vi "Init Runtime.vi"(8 "error in (no error)":errorcluster, 10 "data allocations":T1, 11 "Numeric Limit Compare Config in":refnum<class "Numeric Limit Compare Config.lvclass">) -> (0 "error out":errorcluster, 2 "Skip":bool, 3 "Numeric Limit Compare Config out":refnum<class "Numeric Limit Compare Config.lvclass">)   [LabVIEW 2015, in "Numeric Limit Compare Config.lvclass"]
uses:
  Numeric Limit Compare Config.lvclass
  <vilib>/NI/Tag Bus Module Framework/channel/data tables.ctl
  <vilib>/NI/Tag Bus/dictionary/data dictionary.lvclass
  <vilib>/NI/Tag Bus/dictionary table pair.ctl
  <vilib>/NI/Tag Bus/table/data table.ctl
  Runtime/Numeric Limit Compare.lvclass
  Numeric Limit Compare Config.lvclass/Numeric Limit Compare Config.ctl
  <vilib>/NI/Tag Bus/tag/tag descriptor.lvclass/tag descriptor.ctl
  Runtime/Numeric Limit Compare.lvclass/Numeric Limit Compare.ctl
  Read Channel.vi
  Read Comparison Type.vi
  Read Upper Limit_Limit.vi
  Read Lower Limit.vi
  Read Negate Result.vi
  Read Result Channel.vi
  Runtime/Write Test Value Index.vi
  Runtime/Write Comparison Type.vi
  Runtime/Write Upper limit_limit.vi
  Runtime/Write Lower limit.vi
  Runtime/Write Negate Result.vi
  Runtime/Write Result Index.vi
  <vilib>/NI/Tag Bus/tag/read tag name.vi
  <vilib>/NI/Tag Bus/tag/read data type.vi
  <vilib>/NI/Tag Bus/dictionary/locate tag.vi
  <vilib>/NI/Tag Bus Module Framework/channel/TBM channel.lvclass
  <vilib>/NI/Tag Bus/table/data table.lvlib
  <vilib>/NI/Tag Bus/tag bus.lvlib
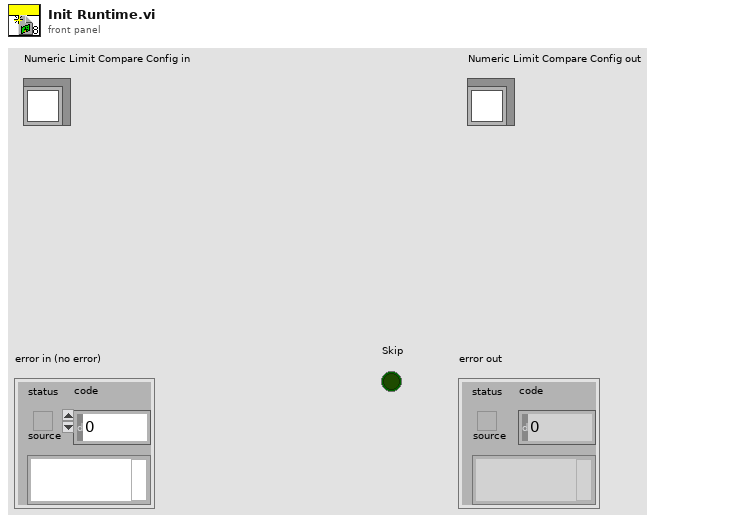
[diagram p1: front panel]
types:
  T1 = typedef "TBM channel.lvclass/data tables.ctl" = cluster{"input data":T2, "processing parameter":T2, "processing result":T2, "output data":T2}
  T2 = typedef "tag bus.lvlib/dictionary table pair.ctl" = cluster{"data dictionary":refnum<class "data dictionary.lvclass">, "data table":T3}
  T3 = typedef "tag bus.lvlib/data table.lvlib/data table.ctl" = cluster{"Double":dbl[], "Single":sgl[], "I64":i64[], "I32":i32[], "I16":i16[], "I8":i8[], "U64":u64[], "U32":u32[], "U16":u16[], "U8":u8[], "Boolean":bool[], "String":string[], "Array of Double":cluster{"DBL Array":dbl[]}[], "Array of Single":cluster{"SGL Array":sgl[]}[], "Array of I64":cluster{"I64 Array":i64[]}[], "Array of I32":cluster{"I32 Array":i32[]}[], "Array of I16":cluster{"I16 Array":i16[]}[], "Array of I8":cluster{"I8 Array":i8[]}[], "Array of U64":cluster{"U64 Array":u64[]}[], "Array of U32":cluster{"U32 Array":u32[]}[], "Array of U16":cluster{"U16 Array":u16[]}[], "Array of U8":cluster{"U8 Array":u8[]}[], "Array of Boolean":cluster{"Boolean Array":bool[]}[], "Array of String":cluster{"String Array":string[]}[]}
  T4 = typedef "Comparison Types.ctl" = enum16{"GELE (>=<=)", "GTLE(><=)", "GTLT(><)", "GELT(>=<)", "EQ(==)", "NE (!=)", "GT(>)", "LT(<)", "GE(>=)", "LE(<=)"}
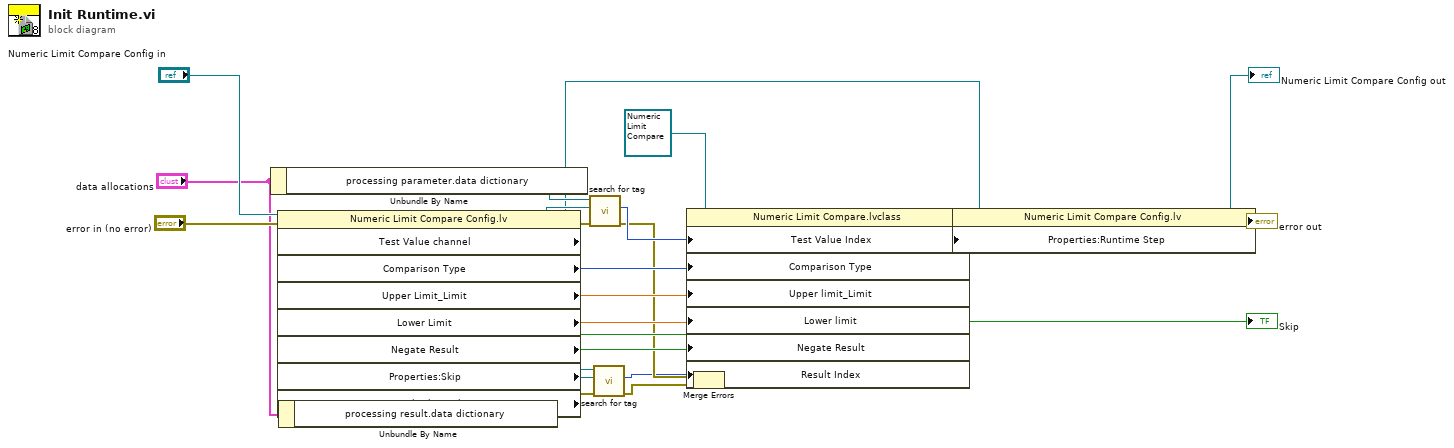
[diagram p0: block diagram]
diagram:
  n1 = Unbundle By Name("data allocations") -> ("processing parameter.data dictionary"=w24:refnum<class "data dictionary.lvclass">)
  n2 = property class="Numeric Limit Compare Config.lv"(reference="Numeric Limit Compare Config in", error in="error in (no error)") -> (reference out=w9:refnum<class "Numeric Limit Compare Config.lvclass">, error out=w5:errorcluster, "Test Value channel"=w22:refnum<class "TBM channel.lvclass">, "Comparison Type"=w19:T4, "Upper Limit_Limit"=w18:dbl, "Lower Limit"=w17:dbl, "Negate Result"=w16:bool, "Properties:Skip"=→"Skip":bool, "Result Channel"=w6:refnum<class "TBM channel.lvclass">)
  n3 = Unbundle By Name("data allocations") -> ("processing result.data dictionary"=w7:refnum<class "data dictionary.lvclass">)
  n4 = call <vilib>:"search for tag.vi"("error in"=w5, "system tag"=w22, "data dictionary in"=w24) -> ("error out"=w3:errorcluster, "index"=w20:i32)  [unwired: 6 in, 1 out]
  n5 = call <vilib>:"search for tag.vi"("error in"=w5, "system tag"=w6, "data dictionary in"=w7) -> ("error out"=w4:errorcluster, "index"=w1:i32)  [unwired: 6 in, 1 out]
  n6 = Merge Errors(w3, w4) -> (w2:errorcluster)
  n7 = property class="Numeric Limit Compare.lvclass"(reference=refnum<class "Numeric Limit Compare.lvclass"> refnum ("Numeric Limit Compare.lvclass"), error in=w2, "Test Value Index"=w20, "Comparison Type"=w19, "Upper limit_Limit"=w18, "Lower limit"=w17, "Negate Result"=w16, "Result Index"=w1) -> (reference out=w12:refnum<class "Numeric Limit Compare.lvclass">, error out=w13:errorcluster)
  n8 = property class="Numeric Limit Compare Config.lv"(reference=w9, error in=w13, "Properties:Runtime Step"=w12) -> (reference out=→"Numeric Limit Compare Config out":refnum<class "Numeric Limit Compare Config.lvclass">, error out=→"error out":errorcluster)
